vi "GroveSensors.vi"() -> ()   [LabVIEW 2016]
uses:
  VIs/uPythonX/uPythonX.xctl
panel:
  in  "Tab Control":T1(tab)=enum."Original Screen"
  in  "Button":T2(xcontrol)={"VISA Refnum in"="ASRL23::INSTR", "Python Code"="import pyb,utime\n\nbutton = pyb.Pin('W16')\n\nbutton()\nutime.sleep(10)\nbutton()\n"}
  in  "Potentiometer":T2(xcontrol)={"VISA Refnum in"="ASRL23::INSTR", "Python Code"="import pyb,utime\n\nadc = pyb.ADC('W24')\n\nwhile True:\n     val = adc.read()\n     print ('%4.2f' % val)\n     utime.sleep_ms(200)\n     "}
  in  "Red Btn":T2(xcontrol)={"VISA Refnum in"="ASRL23::INSTR", "Python Code"="import pyb,utime\n\nBtn = pyb.Pin('Y9', pyb.Pin.IN)\nLED = pyb.Pin('Y10', pyb.Pin.OUT)\n\nBtn.value()\n\ndef btn_callback(line):\n        if LED.value():\n             LED.off()\n        else:\n             LED.on()\n\nBtn_interrupt = pyb.ExtInt(Btn, pyb.ExtInt.IRQ_FALLING, pyb.Pin.PULL_NONE, btn_callback)\n"}
  in  "Relay":T2(xcontrol)={"VISA Refnum in"="ASRL23::INSTR", "Python Code"="import pyb,utime\n\nRelay = pyb.Pin('Y10', pyb.Pin.OUT)\n\nRelay.on()\nutime.sleep_ms(200)\nRelay.off()\n\n"}
  in  "Light Sensor":T2(xcontrol)={"VISA Refnum in"="ASRL23::INSTR", "Python Code"="import pyb,utime\n\nLight = pyb.ADC('W24')\n\nwhile True:\n     Light.read()\n     utime.sleep_ms(200)"}
  in  "VOC":T2(xcontrol)={"VISA Refnum in"="ASRL23::INSTR", "Python Code"="import pyb,utime\n\ni2c = pyb.I2C(2,pyb.I2C.MASTER)\ni2c.scan()\n#should see an 88\n\n#then a lot oof complicated stuff...\n"}
  in  "Ultrasonic":T2(xcontrol)={"VISA Refnum in"="ASRL23::INSTR", "Python Code"="import time\nfrom grove.gpio import GPIO\n\nusleep = lambda x: time.sleep(x / 1000000.0)\n\n_TIMEOUT1 = 1000\n_TIMEOUT2 = 10000\n\nclass GroveUltrasonicRanger(object):\n    def __init__(self, pin):\n        self.dio =GPIO(pin)\n\n    def _get_distance(self):\n        self.dio.dir(GPIO.OUT)\n        self.dio.write(0)\n        usleep(2)\n        self.dio.write(1)\n        usleep(10)\n        self.dio.write(0)\n\n        self.dio.dir(GPIO.IN)\n\n        t0 = time.time()\n        count = 0\n        while count < _TIMEOUT1:\n            if self.dio.read():\n                break\n            count += 1\n        if count >= _TIMEOUT1:\n            return None\n\n        t1 = time.time()\n        count = 0\n        while count < _TIMEOUT2:\n            if not self.dio.read():\n                break\n            count += 1\n        if count >= _TIMEOUT2:\n            return None\n\n        t2 = time.time()\n\n        dt = int((t1 - t0) * 1000000)\n        if dt > 530:\n            return None\n\n        distance = ((t2 - t1) * 1000000 / 29 / 2)    # cm\n\n        return distance\n\n    def get_distance(self):\n        while True:\n            dist = self._get_distance()\n            if dist:\n                return dist\n\nsonar = GroveUltrasonicRanger(int(sys.argv[1]))\n\nprint('Detecting distance...')\nwhile True:\n        print('{} cm'.format(sonar.get_distance()))\n        time.sleep(1)\n"}
  in  "OLED":T2(xcontrol)={"VISA Refnum in"="ASRL23::INSTR", "Python Code"="# http://wiki.seeedstudio.com/Grove-OLED_Display_1.12inch/\n\nimport pyb,utime\n\ni2c = pyb.I2C(2,pyb.I2C.MASTER)\ni2c.scan()\n#should see an 60\n"}
  in  "Motion Detect":T2(xcontrol)={"VISA Refnum in"="ASRL23::INSTR", "Python Code"="# http://wiki.seeedstudio.com/Grove-OLED_Display_1.12inch/\n\nimport pyb,utime\n\nPIR = pyb.Pin('Y9', pyb.Pin.IN)\n\nPIR.value()\n\nwhile True:\n     PIR.value()\n     utime.sleep_ms(200)"}
  in  "Number Display":T2(xcontrol)={"VISA Refnum in"="ASRL23::INSTR", "Python Code"="import  utime\nfrom machine import Pin\n\ncharmap = {\n    '0': 0x3f,\n    '1': 0x06,\n    '2': 0x5b,\n    '3': 0x4f,\n    '4': 0x66,\n    '5': 0x6d,\n    '6': 0x7d,\n    '7': 0x07,\n    '8': 0x7f,\n    '9': 0x6f,\n    'A': 0x77,\n    'B': 0x7f,\n    'b': 0x7C,\n    'C': 0x39,\n    'c': 0x58,\n    'D': 0x3f,\n    'd': 0x5E,\n    'E': 0x79,\n    'F': 0x71,\n    'G': 0x7d,\n    'H': 0x76,\n    'h': 0x74,\n    'I': 0x06,\n    'J': 0x1f,\n    'K': 0x76,\n    'L': 0x38,\n    'l': 0x06,\n    'n': 0x54,\n    'O': 0x3f,\n    'o': 0x5c,\n    'P': 0x73,\n    'r': 0x50,\n    'S': 0x6d,\n    'U': 0x3e,\n    'V': 0x3e,\n    'Y': 0x66,\n    'Z': 0x5b,\n    '-': 0x40,\n    '_': 0x08,\n    ' ': 0x00\n    }\n\nADDR_AUTO = 0x40\nADDR_FIXED = 0x44\nSTARTADDR = 0xC0\nBRIGHT_DARKEST = 0\nBRIGHT_DEFAULT = 2\nBRIGHT_HIGHEST = 7\n\nclass Grove4DigitDisplay(object):\n    colon_index = 1\n\n    def __init__(self, clk, dio, brightness=BRIGHT_DEFAULT):\n        self.brightness = brightness\n\n        self.clk = Pin(clk, Pin.OUT)\n        self.dio = Pin(dio, Pin.OUT)\n        self.data = [0] * 4\n        self.show_colon = False\n\n    def clear(self):\n        self.show_colon = False\n        self.data = [0] * 4\n        self._show()\n\n    def show(self, data):\n        if type(data) is str:\n            for i, c in enumerate(data):\n                if c in charmap:\n                    self.data[i] = charmap[c]\n                else:\n                    self.data[i] = 0\n                if i == self.colon_index and self.show_colon:\n                    self.data[i] |= 0x80\n                if i == 3:\n                    break\n        elif type(data) is int:\n            self.data = [0, 0, 0, charmap['0']]\n            if data < 0:\n                negative = True\n                data = -data\n            else:\n                negative = False\n            index = 3\n            while data != 0:\n                self.data[index] = charmap[str(data % 10)]\n                index -= 1\n                if index < 0:\n                    break\n                data = int(data / 10)\n\n            if negative:\n                if index >= 0:\n                    self.data[index] = charmap['-']\n                else:\n                    self.data = charmap['_'] + [charmap['9']] * 3\n        else:\n            raise ValueError('Not support {}'.format(type(data)))\n        self._show()\n\n    def _show(self):\n        with self:\n            self._transfer(ADDR_AUTO)\n\n        with self:\n            self._transfer(STARTADDR)\n            for i in range(4):\n                self._transfer(self.data[i])\n\n        with self:\n            self._transfer(0x88 + self.brightness)\n\n    def update(self, index, value):\n        if index < 0 or index > 4:\n            return\n\n        if value in charmap:\n            self.data[index] = charmap[value]\n        else:\n            self.data[index] = 0\n\n        if index == self.colon_index and self.show_colon:\n            self.data[index] |= 0x80\n\n        with self:\n            self._transfer(ADDR_FIXED)\n\n        with self:\n            self._transfer(STARTADDR | index)\n            self._transfer(self.data[index])\n\n        with self:\n            self._transfer(0x88 + self.brightness)\n\n\n    def set_brightness(self, brightness):\n        if brightness > 7:\n            brightness = 7\n\n        self.brightness = brightness\n        self._show()\n\n    def set_colon(self, enable):\n        self.show_colon = enable\n        if self.show_colon:\n            self.data[self.colon_index] |= 0x80\n        else:\n            self.data[self.colon_index] &= 0x7F\n        self._show()\n\n    def _transfer(self, data):\n        for _ in range(8):\n            self.clk.value(0)\n            if data & 0x01:\n                self.dio.value(1)\n            else:\n                self.dio.value(0)\n            data >>= 1\n            utime.sleep_us(1)\n            self.clk.value(1)\n            utime.sleep_us(1)\n\n        self.clk.value(0)\n        self.dio.value(1)\n        self.clk.value(1)\n        self.dio.mode(Pin.IN)\n\n        while self.dio.value():\n            utime.sleep_ms(1)\n            if self.dio.value():\n                self.dio.mode(Pin.OUT)\n                self.dio.value(0)\n                self.dio.mode(Pin.IN)\n        self.dio.mode(Pin.OUT)\n\n    def _start(self):\n        self.clk.value(1)\n        self.dio.value(1)\n        self.dio.value(0)\n        self.clk.value(0)\n\n    def _stop(self):\n        self.clk.value(0)\n        self.dio.value(0)\n        self.clk.value(1)\n        self.dio.value(1)\n\n    def __enter__(self):\n        self._start()\n\n    def __exit__(self, exc_type, exc_val, exc_tb):\n        self._stop()\n\ndisplay = Grove4DigitDisplay(clk = 'Y9',dio = 'Y10')\n\ncount = 0\nwhile True:\n     t = (\"%H%M\", utime.localtime(utime.time()))\n     display.show('0701')\n     display.set_colon(count & 1)\n     count += 1\n     utime.sleep(1)\n"}
  in  "LCD":T2(xcontrol)={"VISA Refnum in"="ASRL23::INSTR", "Python Code"="from machine import I2C\nimport utime\n\ni2c = I2C(2)  \ni2c.scan()\n\nTEXT_ADDR = 0x3E   #62\nRGB_ADDR = 0x62    #98\n\ndef setRGB(r,g,b):\n    i2c.writeto_mem(RGB_ADDR, 0x00,b'\\x00')\n    i2c.writeto_mem(RGB_ADDR, 0x01,b'\\x00')\n    i2c.writeto_mem(RGB_ADDR, 0x08,b'\\xAA')\n    i2c.writeto_mem(RGB_ADDR, 0x04, chr(r))\n    i2c.writeto_mem(RGB_ADDR, 0x03,  chr(g))\n    i2c.writeto_mem(RGB_ADDR, 0x02,  chr(b))\n\ndef textCommand(cmd):\n    i2c.writeto_mem(TEXT_ADDR, 0x80, chr(cmd)) #byte out, slave addr, starting memory location on slave\n\ndef setText(text):\n    textCommand(0x02)   # 1 = clear display 2 = reset cursor to home\n    utime.sleep_ms(50)\n    textCommand(0x08 | 0x04) # display on, no cursor\n    textCommand(0x28) # 2 lines\n    utime.sleep_ms(50)\n    count = 0\n    row = 0\n     #  makes it so you do not need to reset the screen\n    while len(text) < 32: # clears the rest of the screen\n        text += \" \" \n    #\n    for c in text:\n        if c == \"\\n\" or count == 16:\n            count = 0\n            row += 1\n            if row == 2:\n                break \n            textCommand(0xC0)\n            if c == \"\\n\":\n                 continue\n            count += 1\n        i2c.writeto_mem(TEXT_ADDR, 0x40,c)\n\nsetRGB(0,255,0)\nsetText(\"Hi \\nKim\")"}
  in  "LCD Ex":T2(xcontrol)={"VISA Refnum in"="ASRL23::INSTR", "Python Code"="from pyb import I2C\nimport utime\n\ni2c = I2C(1, I2C.MASTER)  \n\n\nTEXT_ADDR = 0x3e\nRGB_ADDR = 0x62\n\ndef setRGB(r,g,b):\n    i2c.mem_write(0x00, RGB_ADDR, 0x00)\n    i2c.mem_write(0x00, RGB_ADDR, 0x01)\n    i2c.mem_write(0xAA, RGB_ADDR, 0x08)\n    i2c.mem_write(r, RGB_ADDR, 0x04)\n    i2c.mem_write(g, RGB_ADDR, 0x03)\n    i2c.mem_write(b, RGB_ADDR, 0x02)\n\ndef textCommand(cmd):\n    i2c.mem_write(cmd, TEXT_ADDR, 0x80) #byte out, slave addr, starting memory location on slave\n\ndef setText(text):\n    textCommand(0x02)   # 1 = clear display 2 = reset cursor to home\n    utime.sleep_ms(50)\n    textCommand(0x08 | 0x04) # display on, no cursor\n    textCommand(0x28) # 2 lines\n    utime.sleep_ms(50)\n    count = 0\n    row = 0\n#  makes it so you do not need to reset the screen\n    while len(text) < 32: # clears the rest of the screen\n        text += \" \" \n#\n    for c in text:\n        if c == \"\\n\" or count == 16:\n            count = 0\n            row += 1\n            if row == 2:\n                break\n            textCommand(0xC0)\n            if c == \"\\n\":\n                continue\n        count += 1\n        i2c.mem_write(ord(c), TEXT_ADDR, 0x40)\n\nsetRGB(0,255,0)\nsetText(\"Hi \\nKim\")"}
  # "R"
  # "W"
  # "B"
  # "Y"
  # "R"
  # "W"
  # "B"
  # "Y"
  # "R"
  # "W"
  # "B"
  # "B"
  # "R"
  # "Y - SCL"
  # "W - SDA"
  # "Not working"
  # "B"
  # "R"
  # "Y - SCL"
  # "W - SDA"
  # "Still not working"
  # "B"
  # "R"
  # "W - SDA"
  # "Y - SCL"
  # "Still not working"
  # "B"
  # "R"
  # "W - SDA"
  # "Y - SCL"
  # "Seems to be usually 1..."
  # "Needs translation"
  # "R..power"
  # "B.. grnd"
  # "W.. SDA"
  # "Y.. SCL"
  # "Needs translation"
  # "R..power"
  # "B.. grnd"
  # "W.. SDA"
  # "Y.. SCL"
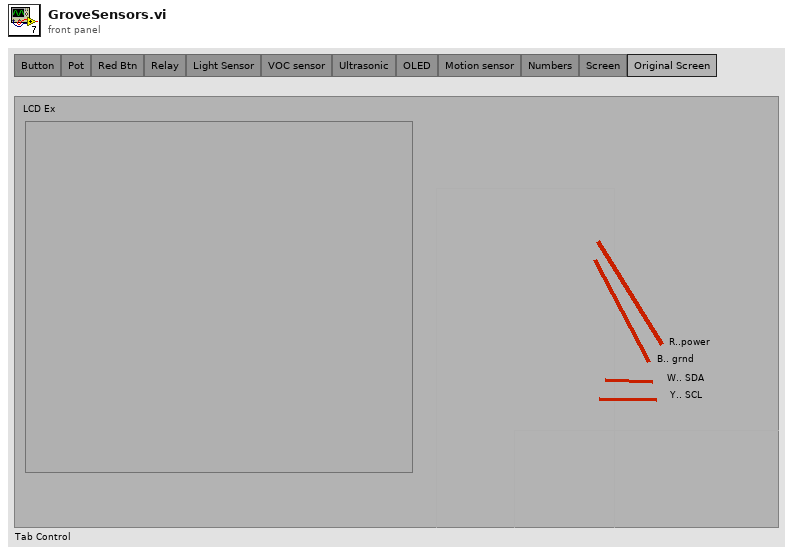
[diagram p1: front panel]
types:
  T1 = enum32{"Button", "Pot", "Red Btn", "Relay", "Light Sensor", "VOC sensor", "Ultrasonic", "OLED", "Motion sensor", "Numbers", "Screen", "Original Screen"}
  T2 = cluster{"VISA Refnum in":refnum<visa-resource-name>, "Python Code":string}
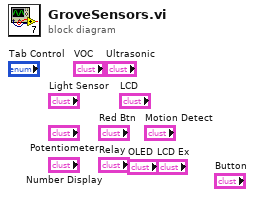
[diagram p0: block diagram]
diagram:
